vi "QRCode VISA Global.vi"() -> ()   [LabVIEW 2026]
panel:
  out "Barcode VISA Global":refnum<visa-resource-name>
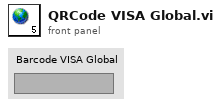
[diagram p1: front panel]
diagram:
